vi "Lab Panel V5.40.vi"() -> ()   [LabVIEW 2017] (continued)
                N: 3 -> [_]
                w247 = TRUE
                n191 = local read "Simulate"() -> (w209:bool)
                n192 = local write "Temp read loop"(0) -> ()
                n193 = case shown="True" w209 {
                  frame False {
                  }
                  frame True {
                    w249 = 20
                    n194 = local write "Ambient Volts"(2.92) -> ()
                    n195 = global write "Global display 3.vi" "Ref deg C"(w249) -> ()
                    n196 = local write "Ref deg C"(w249) -> ()
                  }
                }
                n197 = call "sub vi - GET ALL TEMP v7.vi"("LA01-EN"=w247, "simulate"=w209, "LA02-EN"=w247, "LA03-EN"=w247, "LA04-EN"=w247, "LA05-EN"=w247, "Gen Cal Value"=1) -> ("ID"=w208:T26, "LA01 TEMP"=w245:T27, "LA02 TEMP"=w238:T27, "LA03 TEMP"=w231:T27, "LA04 TEMP"=w224:T27, "LA05 TEMP"=w217:T27)  [unwired: 1 in, 2 out]
                n198 = local write "LAB05 TEMP"(w217) -> ()
                n199 = local write "LAB04 TEMP"(w224) -> ()
                n200 = Unbundle(w231) -> ("T1"=w228:dbl, "T2"=w227:dbl, "T3"=w226:dbl, "T4"=w225:dbl)  [unwired: 2 out]
                n201 = Unbundle(w245) -> ("T1"=w243:dbl, "T2"=w242:dbl, "T3"=w241:dbl, "T4"=w240:dbl)  [unwired: 2 out]
                n202 = Unbundle(w238) -> ("T1"=w235:dbl, "T2"=w234:dbl, "T3"=w233:dbl, "T4"=w232:dbl)  [unwired: 2 out]
                n203 = Unbundle(w224) -> ("T1"=w222:dbl, "T2"=w221:dbl, "T3"=w220:dbl, "T4"=w219:dbl)  [unwired: 2 out]
                n204 = Unbundle(w217) -> ("T1"=w215:dbl, "T2"=w214:dbl, "T3"=w213:dbl, "T4"=w212:dbl)  [unwired: 2 out]
                n205 = local write "LAB01 TEMP"(w245) -> ()
                n206 = local write "LAB02 TEMP"(w238) -> ()
                n207 = local write "LAB03 TEMP"(w231) -> ()
                n208 = Unbundle(w208) -> ("id1"=→"LAB01-TP":bool, "id2"=→"LAB02-TP":bool, "id3"=→"LAB03-TP":bool, "id4"=→"LAB04-TP":bool, "id5"=→"LAB05-TP":bool)
                n209 = local read "TEMP LA05"() -> (w216:T10)
                n210 = local read "TEMP LA04"() -> (w223:T10)
                n211 = local read "TEMP LA02"() -> (w237:T10)
                n212 = local read "TEMP LA03"() -> (w230:T10)
                n213 = local read "TEMP LA01"() -> (w244:T10)
                n214 = Bundle(cluster=w230, "TL-1"=w228, "TN-1"=w227, "TL-2"=w226, "TN-2"=w225) -> (w229:T10)  [unwired: 4 in]
                n215 = Bundle(cluster=w244, "TL-1"=w243, "TN-1"=w242, "TL-2"=w241, "TN-2"=w240) -> (w239:T10)  [unwired: 4 in]
                n216 = Bundle(cluster=w237, "TL-1"=w235, "TN-1"=w234, "TL-2"=w233, "TN-2"=w232) -> (w236:T10)  [unwired: 4 in]
                n217 = Bundle(cluster=w223, "TL-1"=w222, "TN-1"=w221, "TL-2"=w220, "TN-2"=w219) -> (w218:T10)  [unwired: 4 in]
                n218 = Bundle(cluster=w216, "TL-1"=w215, "TN-1"=w214, "TL-2"=w213, "TN-2"=w212) -> (w211:T10)  [unwired: 4 in]
                n219 = local write "TEMP LA03"(w229) -> ()
                n220 = local write "TEMP LA01"(w239) -> ()
                n221 = local write "TEMP LA02"(w236) -> ()
                n222 = local write "TEMP LA05"(w211) -> ()
                n223 = local write "TEMP LA04"(w218) -> ()
              }
            }
            frame #2 {
              w258 = 0
              n224 = local read "LAB01 TEMP"() -> (w260:T13)
              n225 = local read "SIG LAB01-2"() -> (w255:T2)
              n226 = Unbundle By Name(w260) -> ("T1 Live"=w253:dbl, "T1 Neut"=w252:dbl, "T2 Live"=w251:dbl, "T2 Neut"=w250:dbl)  [unwired: 2 out]
              n227 = local read "SIG LAB01-1"() -> (w257:T2)
              n228 = local read "TEMP LA01"() -> (w261:T10)
              n229 = Bundle By Name(cluster=w261, "TL-1"=w253, "TN-1"=w252, "TL-2"=w251, "TN-2"=w250, "TL -1COUNT"=w258, "TN-1 COUNT"=w258, "TL-2 COUNT"=w258, "TN-2 COUNT"=w258) -> (w259:T10)
              n230 = Bundle(cluster=w257, "Tmp Live"=w253, "Tmp Neut"=w252) -> (w256:T2)  [unwired: 3 in]
              n231 = Bundle(cluster=w255, "Tmp Live"=w251, "Tmp Neut"=w250) -> (w254:T2)  [unwired: 3 in]
              n232 = local write "SIG LAB01-2"(w254) -> ()
              n233 = local write "SIG LAB01-1"(w256) -> ()
              n234 = local write "TEMP LA01"(w259) -> ()
            }
            frame #3 {
              w270 = 0
              n235 = local read "LAB02 TEMP"() -> (w272:T13)
              n236 = Unbundle By Name(w272) -> ("T1 Live"=w265:dbl, "T1 Neut"=w264:dbl, "T2 Live"=w263:dbl, "T2 Neut"=w262:dbl)  [unwired: 2 out]
              n237 = local read "SIG LAB02-1"() -> (w269:T2)
              n238 = local read "SIG LAB02-2"() -> (w268:T2)
              n239 = local read "TEMP LA02"() -> (w273:T10)
              n240 = Bundle By Name(cluster=w273, "TL-1"=w265, "TN-1"=w264, "TL-2"=w263, "TN-2"=w262, "TL -1COUNT"=w270, "TN-1 COUNT"=w270, "TL-2 COUNT"=w270, "TN-2 COUNT"=w270) -> (w271:T10)
              n241 = Bundle(cluster=w268, "Tmp Live"=w263, "Tmp Neut"=w262) -> (w266:T2)  [unwired: 3 in]
              n242 = Bundle(cluster=w269, "Tmp Live"=w265, "Tmp Neut"=w264) -> (w267:T2)  [unwired: 3 in]
              n243 = local write "TEMP LA02"(w271) -> ()
              n244 = local write "SIG LAB02-1"(w267) -> ()
              n245 = local write "SIG LAB02-2"(w266) -> ()
            }
            frame #4 {
              w282 = 0
              n246 = local read "LAB03 TEMP"() -> (w284:T13)
              n247 = Unbundle By Name(w284) -> ("T1 Live"=w277:dbl, "T1 Neut"=w276:dbl, "T2 Live"=w275:dbl, "T2 Neut"=w274:dbl)  [unwired: 2 out]
              n248 = local read "SIG LAB03-1"() -> (w281:T2)
              n249 = local read "SIG LAB03-2"() -> (w280:T2)
              n250 = local read "TEMP LA03"() -> (w285:T10)
              n251 = Bundle By Name(cluster=w285, "TL-1"=w277, "TN-1"=w276, "TL-2"=w275, "TN-2"=w274, "TL -1COUNT"=w282, "TN-1 COUNT"=w282, "TL-2 COUNT"=w282, "TN-2 COUNT"=w282) -> (w283:T10)
              n252 = Bundle(cluster=w280, "Tmp Live"=w275, "Tmp Neut"=w274) -> (w278:T2)  [unwired: 3 in]
              n253 = Bundle(cluster=w281, "Tmp Live"=w277, "Tmp Neut"=w276) -> (w279:T2)  [unwired: 3 in]
              n254 = local write "TEMP LA03"(w283) -> ()
              n255 = local write "SIG LAB03-2"(w278) -> ()
              n256 = local write "SIG LAB03-1"(w279) -> ()
            }
            frame #5 {
              w294 = 0
              n257 = local read "LAB04 TEMP"() -> (w296:T13)
              n258 = Unbundle By Name(w296) -> ("T1 Live"=w289:dbl, "T1 Neut"=w288:dbl, "T2 Live"=w287:dbl, "T2 Neut"=w286:dbl)  [unwired: 2 out]
              n259 = local read "SIG LAB04-2"() -> (w292:T2)
              n260 = local read "SIG LAB04-1"() -> (w293:T2)
              n261 = local read "TEMP LA04"() -> (w297:T10)
              n262 = Bundle By Name(cluster=w297, "TL-1"=w289, "TN-1"=w288, "TL-2"=w287, "TN-2"=w286, "TL -1COUNT"=w294, "TN-1 COUNT"=w294, "TL-2 COUNT"=w294, "TN-2 COUNT"=w294) -> (w295:T10)
              n263 = Bundle(cluster=w292, "Tmp Live"=w287, "Tmp Neut"=w286) -> (w290:T2)  [unwired: 3 in]
              n264 = Bundle(cluster=w293, "Tmp Live"=w289, "Tmp Neut"=w288) -> (w291:T2)  [unwired: 3 in]
              n265 = local write "SIG LAB04-2"(w290) -> ()
              n266 = local write "TEMP LA04"(w295) -> ()
              n267 = local write "SIG LAB04-1"(w291) -> ()
            }
            frame #6 {
              w306 = 0
              n268 = local read "LAB05 TEMP"() -> (w308:T13)
              n269 = Unbundle By Name(w308) -> ("T1 Live"=w301:dbl, "T1 Neut"=w300:dbl, "T2 Live"=w299:dbl, "T2 Neut"=w298:dbl)  [unwired: 2 out]
              n270 = local read "SIG LAB05-2"() -> (w304:T2)
              n271 = local read "SIG LAB05-1"() -> (w305:T2)
              n272 = local read "TEMP LA05"() -> (w309:T10)
              n273 = Bundle By Name(cluster=w309, "TL-1"=w301, "TN-1"=w300, "TL-2"=w299, "TN-2"=w298, "TL -1COUNT"=w306, "TN-1 COUNT"=w306, "TL-2 COUNT"=w306, "TN-2 COUNT"=w306) -> (w307:T10)
              n274 = Bundle(cluster=w304, "Tmp Live"=w299, "Tmp Neut"=w298) -> (w302:T2)  [unwired: 3 in]
              n275 = Bundle(cluster=w305, "Tmp Live"=w301, "Tmp Neut"=w300) -> (w303:T2)  [unwired: 3 in]
              n276 = local write "SIG LAB05-2"(w302) -> ()
              n277 = local write "SIG LAB05-1"(w303) -> ()
              n278 = local write "TEMP LA05"(w307) -> ()
            }
          }
        }
        frame #11 {
          # "Create analog task"
          n279 = local read "Simulate"() -> (w310:bool)
          n280 = case shown="False" w310 {
            frame False {
              n281 = local read "SAMPLES"() -> (w313:dbl)
              n282 = local read "RATE (Hz)"() -> (w314:dbl)
              n283 = call "sub vi - AI USB4704 (3)  Create Task v4.vi"("Rate Hz"=w314, "Samples"=w313) -> ("TASK USB 0"=→"AI Task0":i32, "TASK USB 1"=→"AI Task1":i32, "TASK USB 2"=→"AI Task2":i32, "AI Task Er"=w311:bool)  [unwired: 9 in, 1 out]
              n284 = local write "Reset Error"(w311) -> ()
              "AI Task" <- TRUE
            }
            frame True {
            }
          }
        }
        frame #12 {
          # "Enable front panel, all settings done"
          n285 = property on="Tab Control 2" class="TabCtl (strict)"("DisabledEnum"=T17."Enabled" ("Disabled")) -> ()  [unwired: 2 in, 2 out]
          n286 = property on="Tab Control 2" class="TabCtl (strict)"("Value"=0) -> ()  [unwired: 2 in, 2 out]
        }
        frame #13 {
          n287 = property on="Tab Control 2" class="TabCtl (strict)"("Value"=0) -> ()  [unwired: 2 in, 2 out]
        }
      }
    }
    frame #2 {
      w321 = 250.0
      # "frames that only action on certain cycles, 13, 14, 15, 16, 19, 21"
      # "Main Loop"
      n288 = node-c288(w321) -> (w323:T19)  [unwired: 3 in]
      n289 = timed-loop {
        timing: w323 -> [_]
        timing-out: [_] -> w322
        tunnel: w321 -> [w324]
        i -> [w350]
        stop <- w325 stop-if-true
        n290 = node-c288() -> ()  [unwired: 1 in, 1 out]
        n291 = local read "Resets Done"() -> (w329:dbl)
        n292 = local read "SELECT LAB05-2"() -> (w330:T3)
        n293 = local read "SELECT LAB05-1"() -> (w331:T3)
        n294 = local read "SELECT LAB04-2"() -> (w332:T3)
        n295 = local read "SELECT LAB03-1"() -> (w335:T3)
        n296 = local read "SELECT LAB02-2"() -> (w336:T3)
        n297 = local read "SELECT LAB03-2"() -> (w334:T3)
        n298 = local read "SELECT LAB04-1"() -> (w333:T3)
        n299 = local read "SELECT LAB02-1"() -> (w337:T3)
        n300 = local read "run lab03-2"() -> (w344:bool)
        n301 = local read "run lab04-1"() -> (w343:bool)
        n302 = local read "run lab05-1"() -> (w341:bool)
        n303 = local read "run lab04-2"() -> (w342:bool)
        n304 = local read "run lab05-2"() -> (w340:bool)
        n305 = local read "run lab03-1"() -> (w345:bool)
        n306 = local read "run lab02-2"() -> (w346:bool)
        n307 = local read "SELECT LAB01-1"() -> (w339:T3)
        n308 = local read "SELECT LAB01-2"() -> (w338:T3)
        n309 = local read "run lab02-1"() -> (w347:bool)
        n310 = Greater?(x=w329, y=50) -> (0:w326:bool)
        n311 = Or(x=w326, y="stop") -> (x .or. y?=w325:bool)
        n312 = local read "run lab01-1"() -> (w349:bool)
        n313 = local read "run lab01-2"() -> (w348:bool)
        n314 = global write "Global display 1.vi" "stop disp"(w325) -> ()
        n315 = stacked-sequence {
          seq-local: [_ _ w436 _ _ _ _ _ _ _ _ _ _ _ _ _ _ _ _ _ _ _ _ _ _] -> [_ _ _ _ _ _ w2537 _ _ _ _ _ _ _ _ _ _ _ _ _ _ _ _ _ _]
          seq-local: [_ _ w435 _ _ _ _ _ _ _ _ _ _ _ _ _ _ _ _ _ _ _ _ _ _] -> [_ _ _ _ _ _ w2536 _ _ _ _ _ _ _ _ _ _ _ _ _ _ _ _ _ _]
          seq-local: [_ _ w422 _ _ _ _ _ _ _ _ _ _ _ _ _ _ _ _ _ _ _ _ _ _] -> [_ _ _ _ _ _ w2535 _ _ _ _ _ _ _ _ _ _ _ _ _ _ _ _ _ _]
          seq-local: [_ _ w421 _ _ _ _ _ _ _ _ _ _ _ _ _ _ _ _ _ _ _ _ _ _] -> [_ _ _ _ _ _ w2534 _ _ _ _ _ _ _ _ _ _ _ _ _ _ _ _ _ _]
          seq-local: [_ _ w420 _ _ _ _ _ _ _ _ _ _ _ _ _ _ _ _ _ _ _ _ _ _] -> [_ _ _ _ _ _ w2533 _ _ _ _ _ _ _ _ _ _ _ _ _ _ _ _ _ _]
          seq-local: [_ _ w419 _ _ _ _ _ _ _ _ _ _ _ _ _ _ _ _ _ _ _ _ _ _] -> [_ _ _ _ _ _ w2532 _ _ _ _ _ _ _ _ _ _ _ _ _ _ _ _ _ _]
          seq-local: [_ _ w418 _ _ _ _ _ _ _ _ _ _ _ _ _ _ _ _ _ _ _ _ _ _] -> [_ _ _ _ _ _ w2531 _ _ _ _ _ _ _ _ _ _ _ _ _ _ _ _ _ _]
          seq-local: [_ _ w417 _ _ _ _ _ _ _ _ _ _ _ _ _ _ _ _ _ _ _ _ _ _] -> [_ _ _ _ _ _ w2530 _ _ _ _ _ _ _ _ _ _ _ _ _ _ _ _ _ _]
          seq-local: [_ _ w416 _ _ _ _ _ _ _ _ _ _ _ _ _ _ _ _ _ _ _ _ _ _] -> [_ _ _ _ _ _ w2529 _ _ _ _ _ _ _ _ _ _ _ _ _ _ _ _ _ _]
          seq-local: [_ _ w415 _ _ _ _ _ _ _ _ _ _ _ _ _ _ _ _ _ _ _ _ _ _] -> [_ _ _ _ _ _ w2528 _ _ _ _ _ _ _ _ _ _ _ _ _ _ _ _ _ _]
          seq-local: [_ _ _ _ _ _ _ _ _ _ _ _ w3672 _ _ _ _ _ _ _ _ _ _ _ _] -> [_ _ _ _ _ _ _ _ _ _ _ _ _ w3704 _ _ _ _ _ _ _ _ _ _ _]
          tunnel: w349 -> [_ _ _ w452 w700 w2127 w2557 w2873 w3361 _ _ _ _ _ w3988 _ w4945 _ _ w5236 w5540 w5721 _ _ _]
          tunnel: w348 -> [_ _ _ w451 w698 w2126 w2556 w2874 w3360 _ _ _ _ _ w3987 _ w4943 _ _ w5235 w5539 w5719 _ _ _]
          tunnel: w347 -> [_ _ _ w450 w696 w2125 w2555 w2872 w3359 _ _ _ _ _ w3986 _ w4941 _ _ w5234 w5538 w5718 _ _ _]
          tunnel: w346 -> [_ _ _ w449 w694 w2124 w2554 w2871 w3358 _ _ _ _ _ w3985 _ w4939 _ _ w5233 w5537 w5717 _ _ _]
          tunnel: w345 -> [_ _ _ w448 w692 w2123 w2553 w2870 w3357 _ _ _ _ _ w3984 _ w4937 _ _ w5232 w5536 w5716 _ _ _]
          tunnel: w344 -> [_ _ _ w447 w690 w2122 w2552 w2869 w3356 _ _ _ _ _ w3983 _ w4935 _ _ w5231 w5535 w5715 _ _ _]
          tunnel: w343 -> [_ _ _ w446 w688 w2121 w2551 w2868 w3355 _ _ _ _ _ w3982 _ w4933 _ _ w5230 w5534 w5714 _ _ _]
          tunnel: w342 -> [_ _ _ w445 w686 w2120 w2550 w2867 w3354 _ _ _ _ _ w3981 _ w4931 _ _ w5229 w5533 w5713 _ _ _]
          tunnel: w341 -> [_ _ _ w444 w684 w2119 w2549 w2866 w3353 _ _ _ _ _ w3980 _ w4929 _ _ w5228 w5532 w5712 _ _ _]
          tunnel: w340 -> [_ _ _ w443 w682 w2118 w2548 w2865 w3352 _ _ _ _ _ w3979 _ w4927 _ _ w5227 w5531 w5711 _ _ _]
          tunnel: w339 -> [_ _ _ _ w699 w2117 w2547 _ _ _ _ _ _ _ _ _ w4947 _ _ _ _ _ w6182 _ _]
          tunnel: w338 -> [_ _ _ _ w697 w2116 w2546 _ _ _ _ _ _ _ _ _ w4942 _ _ _ _ _ w6181 _ _]
          tunnel: w337 -> [_ _ _ _ w695 w2115 w2545 _ _ _ _ _ _ _ _ _ w4940 _ _ _ _ _ w6180 _ _]
          tunnel: w336 -> [_ _ _ _ w693 w2114 w2544 _ _ _ _ _ _ _ _ _ w4938 _ _ _ _ _ w6179 _ _]
          tunnel: w335 -> [_ _ _ _ w691 w2113 w2543 _ _ _ _ _ _ _ _ _ w4936 _ _ _ _ _ w6178 _ _]
          tunnel: w334 -> [_ _ _ _ w689 w2112 w2542 _ _ _ _ _ _ _ _ _ w4934 _ _ _ _ _ w6177 _ _]
          tunnel: w333 -> [_ _ _ _ w687 w2111 w2541 _ _ _ _ _ _ _ _ _ w4932 _ _ _ _ _ w6176 _ _]
          tunnel: w332 -> [_ _ _ _ w685 w2110 w2540 _ _ _ _ _ _ _ _ _ w4930 _ _ _ _ _ w6175 _ _]
          tunnel: w331 -> [_ _ _ _ w683 w2109 w2539 _ _ _ _ _ _ _ _ _ w4928 _ _ _ _ _ w6174 _ _]
          tunnel: w330 -> [_ _ _ _ w681 w2108 w2538 _ _ _ _ _ _ _ _ _ w4926 _ _ _ _ _ w6173 _ _]
          tunnel: w326 -> [_ _ _ _ _ _ _ _ _ _ _ _ _ _ _ _ _ _ _ _ _ _ _ _ w6285]
          tunnel: w325 -> [_ _ _ _ _ _ _ _ _ _ _ _ _ _ _ _ _ _ _ _ _ _ _ _ w6284]
          tunnel: w324 -> [_ w372 _ _ _ _ _ _ _ _ _ _ _ _ _ _ _ _ _ _ _ _ _ _ _]
          frame #0 {
            n316 = local read "AI Task"() -> (w355:bool)
            n317 = global write "Global 1.vi" "RATE(Hz)"("RATE (Hz)") -> ()
            n318 = case shown="True" w355 {
              frame False {
              }
              frame True {
                n319 = local read "SAMPLES"() -> (w362:dbl)
                n320 = local read "AI Task2"() -> (w368:dbl)
                n321 = local read "AI Task1"() -> (w369:dbl)
                n322 = local read "AI Task0"() -> (w370:dbl)
                n323 = call "sub vi - AI USB4704 (3) v73.vi"("Task0"=w370, "Task1"=w369, "Task2"=w368, "SAMPLES"=w362) -> ("data 0"=→"AI data 0" →"AI Data 0":waveform(dbl)[], "data 1"=→"AI data 1" →"AI Data 1":waveform(dbl)[], "data 2"=→"AI data 2" →"AI Data 2":waveform(dbl)[], "loop time"=→"AI loop time":dbl, "error array"=→"AI Error":errorcluster[])  [unwired: 7 in]
              }
            }
            n324 = call <userlib>:"Periodic Trigger__ogtk.vi"("time (ms)"=u32 1000) -> ("Triggered"=w354:bool)  [unwired: 12 in, 2 out]
            n325 = case shown="True" w354 {
              frame False {
              }
              frame True {
                n326 = control-ref of="This VI"() -> (w361:refnum<vi>)
                n327 = invoke class="VI" method="FP.Get Image"(reference=w361) -> ("image data"=w360:T28)  [unwired: 5 in, 5 out]
                n328 = Build Path(base path="path to JPEG file", name or relative path="FP.jpg") -> (appended path=w357:path)
                n329 = call <vilib>:"Write JPEG File.vi"("image data"=w360, "path to JPEG file"=w357) -> ()  [unwired: 8 in, 2 out]
              }
            }
          }
          frame #1 {
            w379 = FALSE
            # "Loop time (s)"
            # "set up cycle control"
            n330 = local read "jig cycle"() -> (w383:dbl)
            n331 = local read "Amps Fail level"() -> (w377:dbl)
            n332 = local read "Simulate"() -> (w374:bool)
            n333 = Divide(x=w372, y=1000.0) -> (x/y=w371:dbl)
            n334 = Divide(x="JIG ON TIME (S)", y=w371) -> (x/y=→"on loops":dbl)
            n335 = Divide(x="JIG OFF TIME (S)", y=w371) -> (x/y=→"off loops":dbl)
            n336 = Increment(x=w383) -> (x+1=w382:dbl)
            n337 = local write "Simulate IND"(w374) -> ()
            n338 = global write "Global display 3.vi" "Amps Fail"(w377) -> ()
            n339 = local write "TEMP"(w379) -> ()
            n340 = local write "AI"(w379) -> ()
            n341 = local read "Network Directory"() -> (w376:path)
            n342 = local write "jig cycle"(w382) -> ()
            n343 = call "sub vi - check network dir v2.vi"("PATH"=w376) -> ("error"=w375:bool)  [unwired: 10 in]
            n344 = global write "Global display 3.vi" "network drive"(w375) -> ()
            n345 = event shown="[1] \"ADMIN\": Value Change" {
              selector: _ -> [_ _]
              dyn-events: _ -> [_ _]
              timeout: 10 -> [_ _]
              event Timeout {
                n346 = event-data() -> ()  [unwired: 1 in, 3 out]
              }
              event "ADMIN": Value Change {
                n347 = event-data() -> ()  [unwired: 1 in, 6 out]
                n348 = stacked-sequence {
                  seq-local: [_ w387 _] -> [_ _ w388]
                  frame #0 {
                    n349 = global write "Global 1.vi" "password"("9949") -> ()
                  }
                  frame #1 {
                    n350 = call "sub vi - password 1.vi"() -> ("RESULT"=w387:bool)  [unwired: 11 in]
                  }
                  frame #2 {
                    w390 = FALSE
                    n351 = property on="Tab Control 2" class="TabCtl (strict)"() -> ("Pages"=w394:refnum<vi>[])  [unwired: 2 in, 2 out]
                    n352 = Select(t=TRUE, s=w388, f=w390) -> (s? t:f=w389:bool)
                    n353 = Index Array(array=w394, index=8) -> (element=w392:refnum<vi>)
                    n354 = property class="Page"(reference=w392, "PageVis"=w389) -> ()  [unwired: 1 in, 2 out]
                    n355 = local write "ADMIN"(w390) -> ()
                  }
                }
              }
            }
            n356 = local write "network error"(w375) -> ()
          }
          frame #2 {
            w432 = 60.0
            # "Test Cycles"
            # "seconds"
            # "convert temperature rise minutes to cycles"
            n357 = local read "SET LAB05-2"() -> (w396:T5)
            n358 = local read "SET LAB05-1"() -> (w398:T5)
            n359 = local read "SET LAB04-2"() -> (w400:T5)
            n360 = local read "SET LAB01-1"() -> (w414:T6)
            n361 = local read "SET LAB01-2"() -> (w412:T5)
            n362 = local read "SET LAB02-2"() -> (w408:T5)
            n363 = local read "SET LAB04-1"() -> (w402:T5)
            n364 = local read "SET LAB03-1"() -> (w406:T5)
            n365 = local read "SET LAB03-2"() -> (w404:T5)
            n366 = local read "SET LAB02-1"() -> (w410:T5)
            n367 = local read "JIG OFF TIME (S)"() -> (w437:dbl)
            n368 = local read "JIG ON TIME (S)"() -> (w438:dbl)
            n369 = Unbundle By Name(w414) -> ("T-RISE mins"=w413:dbl)
            n370 = Unbundle(w396) -> ("T-RISE mins"=w395:dbl)  [unwired: 4 out]
            n371 = Unbundle(w398) -> ("T-RISE mins"=w397:dbl)  [unwired: 4 out]
            n372 = Unbundle(w400) -> ("T-RISE mins"=w399:dbl)  [unwired: 4 out]
            n373 = Unbundle(w412) -> ("T-RISE mins"=w411:dbl)  [unwired: 4 out]
            n374 = Unbundle(w410) -> ("T-RISE mins"=w409:dbl)  [unwired: 4 out]
            n375 = Unbundle(w402) -> ("T-RISE mins"=w401:dbl)  [unwired: 4 out]
            n376 = Unbundle(w408) -> ("T-RISE mins"=w407:dbl)  [unwired: 4 out]
            n377 = Unbundle(w404) -> ("T-RISE mins"=w403:dbl)  [unwired: 4 out]
            n378 = Unbundle(w406) -> ("T-RISE mins"=w405:dbl)  [unwired: 4 out]
            n379 = Add(x=w438, y=w437) -> (x+y=w431:dbl)
            n380 = Multiply(x=w432, y=w403) -> (x*y=w427:dbl)
            n381 = Multiply(x=w432, y=w401) -> (x*y=w426:dbl)
            n382 = Multiply(x=w432, y=w399) -> (x*y=w425:dbl)
            n383 = Multiply(x=w432, y=w397) -> (x*y=w424:dbl)
            n384 = Multiply(x=w432, y=w395) -> (x*y=w423:dbl)
            n385 = Multiply(x=w432, y=w411) -> (x*y=w433:dbl)
            n386 = Multiply(x=w432, y=w405) -> (x*y=w428:dbl)
            n387 = Multiply(x=w432, y=w413) -> (x*y=w434:dbl)
            n388 = Multiply(x=w432, y=w409) -> (x*y=w430:dbl)
            n389 = Multiply(x=w432, y=w407) -> (x*y=w429:dbl)
            n390 = Divide(x=w424, y=w431) -> (x/y=w416:dbl)
            n391 = Divide(x=w425, y=w431) -> (x/y=w417:dbl)
            n392 = Divide(x=w426, y=w431) -> (x/y=w418:dbl)
            n393 = Divide(x=w423, y=w431) -> (x/y=w415:dbl)
            n394 = Divide(x=w428, y=w431) -> (x/y=w420:dbl)
            n395 = Divide(x=w434, y=w431) -> (x/y=w436:dbl)
            n396 = Divide(x=w433, y=w431) -> (x/y=w435:dbl)
            n397 = Divide(x=w430, y=w431) -> (x/y=w422:dbl)
            n398 = Divide(x=w429, y=w431) -> (x/y=w421:dbl)
            n399 = Divide(x=w427, y=w431) -> (x/y=w419:dbl)
          }
          frame #3 {
            # "control cycle loops"
            n400 = local read "JIG OFF TIME (S)"() -> (w441:dbl)
            n401 = local read "JIG ON TIME (S)"() -> (w440:dbl)
            n402 = local read "on loops"() -> (w456:dbl)
            n403 = local read "off loops"() -> (w455:dbl)
            n404 = local read "jig cycle"() -> (w454:dbl)
            n405 = Add(x=w441, y=w440) -> (x+y=w439:dbl)
            n406 = Add(x=w456, y=w455) -> (x+y=w442:dbl)
            n407 = Greater Or Equal?(x=w454, y=w442) -> (x >= y?=w453:bool)
            n408 = case shown="True" w453 {
              tunnel: w452 -> [_ w490]
              tunnel: w451 -> [_ w489]
              tunnel: w450 -> [_ w488]
              tunnel: w449 -> [_ w487]
              tunnel: w448 -> [_ w486]
              tunnel: w447 -> [_ w485]
              tunnel: w446 -> [_ w484]
              tunnel: w445 -> [_ w483]
              tunnel: w444 -> [_ w482]
              tunnel: w443 -> [_ w481]
              tunnel: w439 -> [_ w480]
              frame False {
              }
              frame True {
                # "increment cycle value and convert cycles to minutes for temp rise"
                n409 = stacked-sequence {
                  frame #0 {
                    n410 = local read "Temp read loop"() -> (w493:dbl)
                    n411 = Increment(x=w493) -> (x+1=w492:dbl)
                    n412 = local write "Temp read loop"(w492) -> ()
                  }
                  frame #1 {
                    n413 = local read "Temp read loop"() -> (w494:dbl)
                    n414 = Greater?(x=w494, y=20) -> (0:w496:bool)
                    n415 = case shown="True" w496 {
                      frame False {
                      }
                      frame True {
                        n416 = local write "Temp read loop"(1) -> ()
                      }
                    }
                  }
                }
                n417 = local read "JIG RELAY CYCLES"() -> (w479:T9)
                n418 = local read "Temp read loop"() -> (→"Tp Up":dbl)
                n419 = Unbundle By Name(w479) -> ("LAB01-1"=w477:dbl, "LAB01-2"=w475:dbl, "LAB02-1"=w473:dbl, "LAB02-2"=w471:dbl, "LAB03-1"=w469:dbl, "LAB03-2"=w467:dbl, "LAB04-1"=w465:dbl, "LAB04-2"=w463:dbl, "LAB05-1"=w461:dbl, "LAB05-2"=w459:dbl)
                n420 = stacked-sequence {
                  tunnel: w490 -> [w508 _ _ _ _ _ _ _ _ _]
                  tunnel: w489 -> [_ w525 _ _ _ _ _ _ _ _]
                  tunnel: w488 -> [_ _ w542 _ _ _ _ _ _ _]
                  tunnel: w487 -> [_ _ _ w559 _ _ _ _ _ _]
                  tunnel: w486 -> [_ _ _ _ w576 _ _ _ _ _]
                  tunnel: w485 -> [_ _ _ _ _ w593 _ _ _ _]
                  tunnel: w484 -> [_ _ _ _ _ _ w610 _ _ _]
                  tunnel: w483 -> [_ _ _ _ _ _ _ w627 _ _]
                  tunnel: w482 -> [_ _ _ _ _ _ _ _ w644 _]
                  tunnel: w481 -> [_ _ _ _ _ _ _ _ _ w661]
                  tunnel: w480 -> [w505 w522 w539 w556 w573 w590 w607 w624 w641 w658]
                  tunnel: w477 -> [w499 _ _ _ _ _ _ _ _ _]
                  tunnel: [w498 _ _ _ _ _ _ _ _ _] -> w476
                  tunnel: w475 -> [_ w516 _ _ _ _ _ _ _ _]
                  tunnel: [_ w515 _ _ _ _ _ _ _ _] -> w474
                  tunnel: w473 -> [_ _ w533 _ _ _ _ _ _ _]
                  tunnel: [_ _ w532 _ _ _ _ _ _ _] -> w472
                  tunnel: w471 -> [_ _ _ w550 _ _ _ _ _ _]
                  tunnel: [_ _ _ w549 _ _ _ _ _ _] -> w470
                  tunnel: w469 -> [_ _ _ _ w567 _ _ _ _ _]
                  tunnel: [_ _ _ _ w566 _ _ _ _ _] -> w468
                  tunnel: w467 -> [_ _ _ _ _ w584 _ _ _ _]
                  tunnel: [_ _ _ _ _ w583 _ _ _ _] -> w466
                  tunnel: w465 -> [_ _ _ _ _ _ w601 _ _ _]
                  tunnel: [_ _ _ _ _ _ w600 _ _ _] -> w464
                  tunnel: w463 -> [_ _ _ _ _ _ _ w618 _ _]
                  tunnel: [_ _ _ _ _ _ _ w617 _ _] -> w462
                  tunnel: w461 -> [_ _ _ _ _ _ _ _ w635 _]
                  tunnel: [_ _ _ _ _ _ _ _ w634 _] -> w460
                  tunnel: w459 -> [_ _ _ _ _ _ _ _ _ w652]
                  tunnel: [_ _ _ _ _ _ _ _ _ w651] -> w458
                  frame #0 {
                    n421 = local read "DISP LAB01-1"() -> (w503:T4)
                    n422 = Unbundle By Name(w503) -> ("CYCLE"=w504:dbl)
                    n423 = case shown="True" w508 {
                      tunnel: w504 -> [w510 w514]
                      tunnel: [w510 w513] -> w502
                      tunnel: w499 -> [w509 w512]
                      tunnel: [w509 w511] -> w498
                      frame False {
                      }
                      frame True {
                        n424 = Increment(x=w512) -> (x+1=w511:dbl)
                        n425 = Increment(x=w514) -> (x+1=w513:dbl)
                      }
                    }
                    n426 = Multiply(x=w502, y=w505) -> (x*y=w506:dbl)
                    n427 = Divide(x=w506, y=60.0) -> (x/y=w501:dbl)
                    n428 = Bundle By Name(cluster=w503, "CYCLE"=w502, "MINS"=w501) -> (w500:T4)
                    n429 = local write "DISP LAB01-1"(w500) -> ()
                  }
                  frame #1 {
                    n430 = local read "DISP LAB01-2"() -> (w520:T4)
                    n431 = Unbundle By Name(w520) -> ("CYCLE"=w521:dbl)
                    n432 = case shown="True" w525 {
                      tunnel: w521 -> [w527 w531]
                      tunnel: [w527 w530] -> w518
                      tunnel: w516 -> [w526 w529]
                      tunnel: [w526 w528] -> w515
                      frame False {
                      }
                      frame True {
                        n433 = Increment(x=w529) -> (x+1=w528:dbl)
                        n434 = Increment(x=w531) -> (x+1=w530:dbl)
                      }
                    }
                    n435 = Multiply(x=w518, y=w522) -> (x*y=w523:dbl)
                    n436 = Divide(x=w523, y=60.0) -> (x/y=w517:dbl)
                    n437 = Bundle By Name(cluster=w520, "CYCLE"=w518, "MINS"=w517) -> (w519:T4)
                    n438 = local write "DISP LAB01-2"(w519) -> ()
                  }
                  frame #2 {
                    n439 = local read "DISP LAB02-1"() -> (w537:T4)
                    n440 = Unbundle By Name(w537) -> ("CYCLE"=w538:dbl)
                    n441 = case shown="True" w542 {
                      tunnel: [w544 w548] -> w535
                      tunnel: w538 -> [w544 w547]
                      tunnel: w533 -> [w543 w546]
                      tunnel: [w543 w545] -> w532
                      frame False {
                      }
                      frame True {
                        n442 = Increment(x=w546) -> (x+1=w545:dbl)
                        n443 = Increment(x=w547) -> (x+1=w548:dbl)
                      }
                    }
                    n444 = Multiply(x=w535, y=w539) -> (x*y=w540:dbl)
                    n445 = Divide(x=w540, y=60.0) -> (x/y=w534:dbl)
                    n446 = Bundle By Name(cluster=w537, "CYCLE"=w535, "MINS"=w534) -> (w536:T4)
                    n447 = local write "DISP LAB02-1"(w536) -> ()
                  }
                  frame #3 {
                    n448 = local read "DISP LAB02-2"() -> (w554:T4)
                    n449 = Unbundle By Name(w554) -> ("CYCLE"=w555:dbl)
                    n450 = case shown="True" w559 {
                      tunnel: [w561 w565] -> w553
                      tunnel: w555 -> [w561 w564]
                      tunnel: w550 -> [w560 w563]
                      tunnel: [w560 w562] -> w549
                      frame False {
                      }
                      frame True {
                        n451 = Increment(x=w563) -> (x+1=w562:dbl)
                        n452 = Increment(x=w564) -> (x+1=w565:dbl)
                      }
                    }
                    n453 = Multiply(x=w553, y=w556) -> (x*y=w557:dbl)
                    n454 = Divide(x=w557, y=60.0) -> (x/y=w552:dbl)
                    n455 = Bundle By Name(cluster=w554, "CYCLE"=w553, "MINS"=w552) -> (w551:T4)
                    n456 = local write "DISP LAB02-2"(w551) -> ()
                  }
                  frame #4 {
                    n457 = local read "DISP LAB03-1"() -> (w571:T4)
                    n458 = Unbundle(w571) -> ("CYCLE"=w572:dbl)  [unwired: 2 out]
                    n459 = case shown="True" w576 {
                      tunnel: [w578 w582] -> w568
                      tunnel: w572 -> [w578 w581]
                      tunnel: w567 -> [w577 w580]
                      tunnel: [w577 w579] -> w566
                      frame False {
                      }
                      frame True {
                        n460 = Increment(x=w580) -> (x+1=w579:dbl)
                        n461 = Increment(x=w581) -> (x+1=w582:dbl)
                      }
                    }
                    n462 = Multiply(x=w568, y=w573) -> (x*y=w574:dbl)
                    n463 = Divide(x=w574, y=60.0) -> (x/y=w569:dbl)
                    n464 = Bundle(cluster=w571, "CYCLE"=w568, "MINS"=w569) -> (w570:T4)  [unwired: 1 in]
                    n465 = local write "DISP LAB03-1"(w570) -> ()
                  }
                  frame #5 {
                    n466 = local read "DISP LAB03-2"() -> (w588:T4)
                    n467 = Unbundle(w588) -> ("CYCLE"=w589:dbl)  [unwired: 2 out]
                    n468 = case shown="True" w593 {
                      tunnel: [w595 w599] -> w587
                      tunnel: w589 -> [w595 w598]
                      tunnel: w584 -> [w594 w597]
                      tunnel: [w594 w596] -> w583
                      frame False {
                      }
                      frame True {
                        n469 = Increment(x=w597) -> (x+1=w596:dbl)
                        n470 = Increment(x=w598) -> (x+1=w599:dbl)
                      }
                    }
                    n471 = Multiply(x=w587, y=w590) -> (x*y=w591:dbl)
                    n472 = Divide(x=w591, y=60.0) -> (x/y=w586:dbl)
                    n473 = Bundle(cluster=w588, "CYCLE"=w587, "MINS"=w586) -> (w585:T4)  [unwired: 1 in]
                    n474 = local write "DISP LAB03-2"(w585) -> ()
                  }
                  frame #6 {
                    n475 = local read "DISP LAB04-1"() -> (w605:T4)
                    n476 = Unbundle(w605) -> ("CYCLE"=w606:dbl)  [unwired: 2 out]
                    n477 = case shown="True" w610 {
                      tunnel: [w612 w616] -> w603
                      tunnel: w606 -> [w612 w615]
                      tunnel: w601 -> [w611 w614]
                      tunnel: [w611 w613] -> w600
                      frame False {
                      }
                      frame True {
                        n478 = Increment(x=w614) -> (x+1=w613:dbl)
                        n479 = Increment(x=w615) -> (x+1=w616:dbl)
                      }
                    }
                    n480 = Multiply(x=w603, y=w607) -> (x*y=w608:dbl)
                    n481 = Divide(x=w608, y=60.0) -> (x/y=w602:dbl)
                    n482 = Bundle(cluster=w605, "CYCLE"=w603, "MINS"=w602) -> (w604:T4)  [unwired: 1 in]
                    n483 = local write "DISP LAB04-1"(w604) -> ()
                  }
                  frame #7 {
                    n484 = local read "DISP LAB04-2"() -> (w622:T4)
                    n485 = Unbundle(w622) -> ("CYCLE"=w623:dbl)  [unwired: 2 out]
                    n486 = case shown="True" w627 {
                      tunnel: [w629 w633] -> w620
                      tunnel: w623 -> [w629 w632]
                      tunnel: w618 -> [w628 w631]
                      tunnel: [w628 w630] -> w617
                      frame False {
                      }
                      frame True {
                        n487 = Increment(x=w631) -> (x+1=w630:dbl)
                        n488 = Increment(x=w632) -> (x+1=w633:dbl)
                      }
                    }
                    n489 = Multiply(x=w620, y=w624) -> (x*y=w626:dbl)
                    n490 = Divide(x=w626, y=60.0) -> (x/y=w619:dbl)
                    n491 = Bundle(cluster=w622, "CYCLE"=w620, "MINS"=w619) -> (w621:T4)  [unwired: 1 in]
                    n492 = local write "DISP LAB04-2"(w621) -> ()
                  }
                  frame #8 {
                    n493 = local read "DISP LAB05-1"() -> (w639:T4)
                    n494 = Unbundle(w639) -> ("CYCLE"=w640:dbl)  [unwired: 2 out]
                    n495 = case shown="True" w644 {
                      tunnel: [w646 w650] -> w637
                      tunnel: w640 -> [w646 w649]
                      tunnel: w635 -> [w645 w648]
                      tunnel: [w645 w647] -> w634
                      frame False {
                      }
                      frame True {
                        n496 = Increment(x=w648) -> (x+1=w647:dbl)
                        n497 = Increment(x=w649) -> (x+1=w650:dbl)
                      }
                    }
                    n498 = Multiply(x=w637, y=w641) -> (x*y=w642:dbl)
                    n499 = Divide(x=w642, y=60.0) -> (x/y=w636:dbl)
                    n500 = Bundle(cluster=w639, "CYCLE"=w637, "MINS"=w636) -> (w638:T4)  [unwired: 1 in]
                    n501 = local write "DISP LAB05-1"(w638) -> ()
                  }
                  frame #9 {
                    n502 = local read "DISP LAB05-2"() -> (w657:T4)
                    n503 = Unbundle(w657) -> ("CYCLE"=w656:dbl)  [unwired: 2 out]
                    n504 = case shown="True" w661 {
                      tunnel: [w663 w667] -> w655
                      tunnel: w656 -> [w663 w666]
                      tunnel: w652 -> [w662 w665]
                      tunnel: [w662 w664] -> w651
                      frame False {
                      }
                      frame True {
                        n505 = Increment(x=w665) -> (x+1=w664:dbl)
                        n506 = Increment(x=w666) -> (x+1=w667:dbl)
                      }
                    }
                    n507 = Multiply(x=w655, y=w658) -> (x*y=w659:dbl)
                    n508 = Divide(x=w659, y=60.0) -> (x/y=w654:dbl)
                    n509 = Bundle(cluster=w657, "CYCLE"=w655, "MINS"=w654) -> (w653:T4)  [unwired: 1 in]
                    n510 = local write "DISP LAB05-2"(w653) -> ()
                  }
                }
                n511 = local write "jig cycle"(0) -> ()
                n512 = Bundle By Name(cluster=w479, "LAB01-1"=w476, "LAB01-2"=w474, "LAB02-1"=w472, "LAB02-2"=w470, "LAB03-1"=w468, "LAB03-2"=w466, "LAB04-1"=w464, "LAB04-2"=w462, "LAB05-1"=w460, "LAB05-2"=w458) -> (w478:T9)
                n513 = local write "JIG RELAY CYCLES"(w478) -> ()
              }
            }
          }
          frame #4 {
            # "Note : Run lab0X-N variables are set which are written to digital I/O in frame 11"
            # "Why are these here?"
            # "START & STOP test RUN switch change, start test if true and stop test if false"
            n514 = Get Date/Time In Seconds() -> (seconds since 1Jan1904=w679:timestamp)
            n515 = local read "C drive data root dir"() -> (w672:path)
            n516 = Format Date/Time String(time format string (%c)="%b\\%a%d", seconds (now)=w679) -> (date/time string=w703:string)  [unwired: 1 in]
            n517 = Format Date/Time String(time format string (%c)="%H%M", seconds (now)=w679) -> (date/time string=w701:string)  [unwired: 1 in]
            n518 = Format Date/Time String(time format string (%c)="LabPanel%Y", seconds (now)=w679) -> (date/time string=w678:string)  [unwired: 1 in]
            n519 = Path To String(path=w672) -> (string=w675:string)
            n520 = global write "Global 1.vi" "C drive root path"(w672) -> ()
            n521 = local read "Ref deg C"() -> (w668:dbl)
            n522 = Concatenate Strings(w675, "\\") -> (w673:string)
            n523 = event shown="[10] \"RUN LAB05-2\": Value Change" {
              selector: _ -> [_ _ _ _ _ _ _ _ _ _ _]
              dyn-events: _ -> [_ _ _ _ _ _ _ _ _ _ _]
              timeout: 10 -> [_ _ _ _ _ _ _ _ _ _ _]
              tunnel: w673 -> [_ w716 w856 w997 w1137 w1277 w1417 w1557 w1697 w1837 w1978]
              tunnel: w703 -> [_ w715 w855 w996 w1136 w1276 w1416 w1556 w1696 w1836 w1977]
              tunnel: w701 -> [_ w713 w854 w995 w1135 w1275 w1415 w1555 w1695 w1835 w1976]
              tunnel: w699 -> [_ w714 _ _ _ _ _ _ _ _ _]
              tunnel: w700 -> [_ _ _ _ _ _ _ _ _ _ _]
              tunnel: w698 -> [_ _ _ _ _ _ _ _ _ _ _]
              tunnel: w697 -> [_ _ w853 _ _ _ _ _ _ _ _]
              tunnel: w696 -> [_ _ _ _ _ _ _ _ _ _ _]
              tunnel: w695 -> [_ _ _ w994 _ _ _ _ _ _ _]
              tunnel: w694 -> [_ _ _ _ _ _ _ _ _ _ _]
              tunnel: w693 -> [_ _ _ _ w1134 _ _ _ _ _ _]
              tunnel: w692 -> [_ _ _ _ _ _ _ _ _ _ _]
              tunnel: w691 -> [_ _ _ _ _ w1274 _ _ _ _ _]
              tunnel: w690 -> [_ _ _ _ _ _ _ _ _ _ _]
              tunnel: w689 -> [_ _ _ _ _ _ w1414 _ _ _ _]
              tunnel: w688 -> [_ _ _ _ _ _ _ _ _ _ _]
              tunnel: w687 -> [_ _ _ _ _ _ _ w1554 _ _ _]
              tunnel: w686 -> [_ _ _ _ _ _ _ _ _ _ _]
              tunnel: w685 -> [_ _ _ _ _ _ _ _ w1694 _ _]
              tunnel: w684 -> [_ _ _ _ _ _ _ _ _ _ _]
              tunnel: w683 -> [_ _ _ _ _ _ _ _ _ w1834 _]
              tunnel: w682 -> [_ _ _ _ _ _ _ _ _ _ _]
              tunnel: w681 -> [_ _ _ _ _ _ _ _ _ _ w1975]
              tunnel: w678 -> [_ w712 w852 w993 w1133 w1273 w1413 w1553 w1693 w1833 w1974]
              tunnel: [_ w711 w851 w992 w1132 w1272 w1412 w1552 w1692 w1832 w1973] -> w676
              tunnel: "RESET CYCLES TO ZERO?" -> [_ w710 w849 w990 w1130 w1270 w1410 w1550 w1690 w1830 w1971]
              tunnel: "YES" -> [_ w709 w848 w989 w1129 w1269 w1409 w1549 w1689 w1829 w1970]
              tunnel: "NO" -> [_ w708 w847 w988 w1128 w1268 w1408 w1548 w1688 w1828 w1969]
              tunnel: w668 -> [_ w705 w846 w986 w1127 w1267 w1407 w1547 w1687 w1827 w1967]
              event Timeout {
                n524 = event-data() -> ()  [unwired: 1 in, 3 out]
              }
              event "RUN LAB01-1": Value Change {
                n525 = event-data() -> ("NewVal"=w706:bool)  [unwired: 1 in, 5 out]
                n526 = local read "SIG LAB01-1"() -> (w707:T2)
                n527 = local write "run lab01-1"(w706) -> ()
                n528 = case shown="False" w706 {
                  tunnel: w716 -> [_ w754]
                  tunnel: w715 -> [_ w753]
                  tunnel: w714 -> [w718 w752]
                  tunnel: w713 -> [_ w751]
                  tunnel: w712 -> [_ w750]
                  tunnel: [w717 w749] -> w711
                  tunnel: w710 -> [_ w748]
                  tunnel: w709 -> [_ w747]
                  tunnel: w708 -> [_ w746]
                  tunnel: w707 -> [_ w745]
                  tunnel: w705 -> [_ w744]
                  frame False {
                    # "stop test"
                    n529 = stacked-sequence {
                      tunnel: w718 -> [_ w730 _]
                      tunnel: [_ w722 _] -> w717
                      frame #0 {
                        n530 = local read "DISP LAB01-1"() -> (w721:T4)
                        n531 = Bundle(cluster=w721, "STATUS"="STOP") -> (w719:T4)  [unwired: 2 in]
                        n532 = local write "DISP LAB01-1"(w719) -> ()
                      }
                      frame #1 {
                        n533 = local read "DISP LAB01-1"() -> (w729:T4)
                        n534 = Unbundle(w729) -> ("CYCLE"=w727:dbl, "MINS"=w728:dbl)  [unwired: 1 out]
                        n535 = case shown="\"CYCLE TEST\"" w730 {
                          tunnel: w728 -> [_ _ w737]
                          tunnel: w727 -> [w735 w736 _]
                          tunnel: [w735 w736 w737] -> w726
                          frame "CHART TEST", Default {
                          }
                          frame "CYCLE TEST" {
                          }
                          frame "T-RISE TEST" {
                          }
                        }
                        n536 = local read "TDMS LAB01-1"() -> (w734:refnum<k34>)
                        n537 = Build Array("STOPPED") -> (w731:string[])
                        n538 = Build Array(w726) -> (w725:dbl[])
                        n539 = TDMS Write(0:w734, 5:"TEST RESULT", 7:w731, 9:w725) -> (4:w723:refnum<k34>, 15:w724:errorcluster)  [unwired: 2 in, 2 out]
                        n540 = TDMS Close(8:w724, 11:w723) -> (0:w722:errorcluster)  [unwired: 1 out]
                      }
                      frame #2 {
                        n541 = stacked-sequence {
                          tunnel: "LAB01-1" -> [w740 w742]
                          frame #0 {
                            n542 = call "sub vi - defrag tdms v1.vi"("panel id"=w740) -> ("error out"=w739:errorcluster)  [unwired: 10 in]
                            n543 = local write "data file error"(w739) -> ()
                          }
                          frame #1 {
                            n544 = call "Save data file (stop) v3.vi"("panel id"=w742) -> ("network file save error"=w741:errorcluster)  [unwired: 9 in, 1 out]
                            n545 = local write "RESULT LAB01-1"(FALSE) -> ()
                            n546 = local write "data file error"(w741) -> ()
                          }
                        }
                      }
                    }
                  }
                  frame True {
                    n547 = stacked-sequence {
                      seq-local: [w756 _] -> [_ w760]
                      tunnel: w754 -> [_ w770]
                      tunnel: w753 -> [_ w769]
                      tunnel: w752 -> [_ w768]
                      tunnel: w751 -> [_ w767]
                      tunnel: w750 -> [_ w766]
                      tunnel: [_ w765] -> w749
                      tunnel: w748 -> [_ w764]
                      tunnel: w747 -> [_ w763]
                      tunnel: w746 -> [_ w762]
                      tunnel: w745 -> [w758 w761]
                      tunnel: w744 -> [_ w759]
                      frame #0 {
                        n548 = Unbundle(w758) -> ("AMPS"=w757:dbl)  [unwired: 4 out]
                        n549 = call "Check For Amps on v1.vi"("ID"="LAB01-1", "amps"=w757) -> ("amps"=w756:bool)  [unwired: 9 in]
                      }
                      frame #1 {
                        n550 = case shown="True" w760 {
                          tunnel: w770 -> [_ w783]
                          tunnel: w769 -> [_ w782]
                          tunnel: w768 -> [_ w781]
                          tunnel: w767 -> [_ w780]
                          tunnel: w766 -> [_ w779]
                          tunnel: [errorcluster {"status"=FALSE, "code"=0, "source"=""} ("error out") w778] -> w765
                          tunnel: w764 -> [_ w777]
                          tunnel: w763 -> [_ w776]
                          tunnel: w762 -> [_ w775]
                          tunnel: w761 -> [_ w774]
                          tunnel: w759 -> [_ w773]
                          frame False {
                            w771 = FALSE
                            n551 = local write "RUN LAB01-1"(w771) -> ()
                            n552 = local write "run lab01-1"(w771) -> ()
                          }
                          frame True {
                            n553 = stacked-sequence {
                              seq-local: [w784 _ _ _ _] -> [_ w805 _ _ _]
                              tunnel: w783 -> [w789 _ _ _ _]
                              tunnel: w782 -> [w785 _ _ _ _]
                              tunnel: w781 -> [w799 _ _ _ _]
                              tunnel: w780 -> [w792 _ _ _ _]
                              tunnel: w779 -> [w787 _ _ _ _]
                              tunnel: [_ w806 _ _ _] -> w778
                              tunnel: w777 -> [_ _ _ w827 _]
                              tunnel: w776 -> [_ _ _ w837 _]
                              tunnel: w775 -> [_ _ _ w836 _]
                              tunnel: w774 -> [_ _ _ _ _]
                              tunnel: w773 -> [_ _ _ _ w843]
                              frame #0 {
                                w786 = "\\"
                                n554 = case shown="\"CHART TEST\", Default" w799 {
                                tunnel: ["L01-1-CHART TEST-" "L01-1-CYCLE TEST-" "L01-1-T-RISE TEST-"] -> w795
                                frame "CHART TEST", Default {
                                }
                                frame "CYCLE TEST" {
                                }
                                frame "T-RISE TEST" {
                                }
                                }
                                n555 = local read "SET LAB01-1"() -> (w794:T6)
                                n556 = Unbundle By Name(w794) -> ("DESCRIPTION"=w793:string)
                                n557 = Concatenate Strings(w789, "\\", w787, w786, w785, w786) -> (w796:string)
                                n558 = String To Path(string=w796) -> (path=w798:path)
                                n559 = Concatenate Strings(w796, w795, w793, "-", w792, ".tdms") -> (w784:string)
                                n560 = Create Folder(path (use dialog)=w798) -> (error out=w797:errorcluster)  [unwired: 2 in, 2 out]
                                n561 = call <vilib>:"Clear Errors.vi"("error in (no error)"=w797) -> ()  [unwired: 5 in, 2 out]
                                n562 = global write "Global 1.vi" "LAB01-1 FILE"(w784) -> ()
                              }
                              frame #1 {
                                (unwired) FALSE
                                n563 = String To Path(string=w805) -> (path=w803:path)
                                n564 = TDMS Open(6:FALSE, 10:T22."create or replace" ("operation (0:open)"), 11:w803) -> (0:w806:errorcluster, 3:→"TDMS LAB01-1":refnum<k34>)  [unwired: 4 in]
                              }
                              frame #2 {
                                n565 = local read "TDMS LAB01-1"() -> (w825:refnum<k34>)
                                n566 = local read "SET LAB01-1"() -> (w814:T6)
                                n567 = Build Array("Testers Name", "Description", "Set Test Cycles", "T-Rise minutes", "T-Rise Deg C") -> (w815:string[])
                                n568 = Unbundle(w814) -> ("NAME"=w813:string, "DESCRIPTION"=w812:string, "CYCLES"=w811:dbl, "T-RISE mins"=w810:dbl, "T-RISE deg C"=w809:dbl)
                                n569 = Number To Decimal String(number=w811) -> (decimal integer string=w824:string)  [unwired: 1 in]
                                n570 = Number To Decimal String(number=w810) -> (decimal integer string=w823:string)  [unwired: 1 in]
                                n571 = Number To Decimal String(number=w809) -> (decimal integer string=w822:string)  [unwired: 1 in]
                                n572 = Build Array(w813, w812, w824, w823, w822) -> (w821:string[])
                                n573 = TDMS Set Properties(5:w821, 7:w815, 11:w825) -> ()  [unwired: 3 in, 4 out]
                              }
                              frame #3 {
                                n574 = local read "DISP LAB01-1"() -> (w835:T4)
                                n575 = Concatenate Strings("LAB01-1  ", w827) -> (w826:string)
                                n576 = Two Button Dialog(message=w826, 1:w836, 2:w837) -> (T button?=w829:bool)
                                n577 = case shown="True" w829 {
                                tunnel: w835 -> [w840 w841]
                                tunnel: [w840 w841] -> w834
                                tunnel: [w839 w842] -> w833
                                tunnel: [w838 w842] -> w832
                                frame False {
                                n578 = Unbundle(w840) -> ("CYCLE"=w839:dbl, "MINS"=w838:dbl)  [unwired: 1 out]
                                }
                                frame True {
                                w842 = 0.0
                                }
                                }
                                n579 = Bundle(cluster=w834, "CYCLE"=w833, "MINS"=w832, "STATUS"="RUN") -> (w831:T4)
                                n580 = local write "DISP LAB01-1"(w831) -> ()
                              }
                              frame #4 {
                                n581 = local read "TEMP START LAB01-1"() -> (w845:cluster{"TL":dbl, "TN":dbl})
                                n582 = Bundle(cluster=w845, "TL"=w843, "TN"=w843) -> (w844:cluster{"TL":dbl, "TN":dbl})
                                n583 = local write "TEMP START LAB01-1"(w844) -> ()
                              }
                            }
